vi "End Time.vi"(4 "Manual # of Averages":i32=1, 5 "Freq Index":i32, 6 "Signal Averages Selection":bool, 7 "Amp Index":i32, 8 "# of Pre-Check Points Collected (above 1 HZ)":i32=10, 9 "Np to Pre-Check (<1Hz)":i32=1, 10 "fp Array":dbl[](array[numeric]), 11 "# Amplitudes":i32) -> (3 "Estimated \nEnd Time":timestamp format="%<%I:%M:%S %p\n%x>T")   [LabVIEW 2018]
panel:
  # "Estimate time that NLEISRun sweep will end"
  # "Input"
  # "Output"
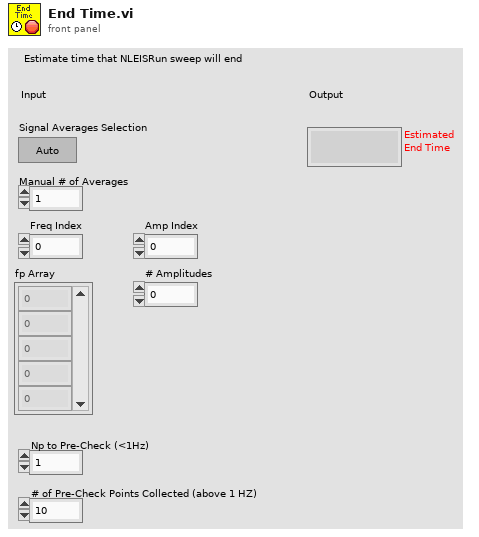
[diagram p1: front panel]
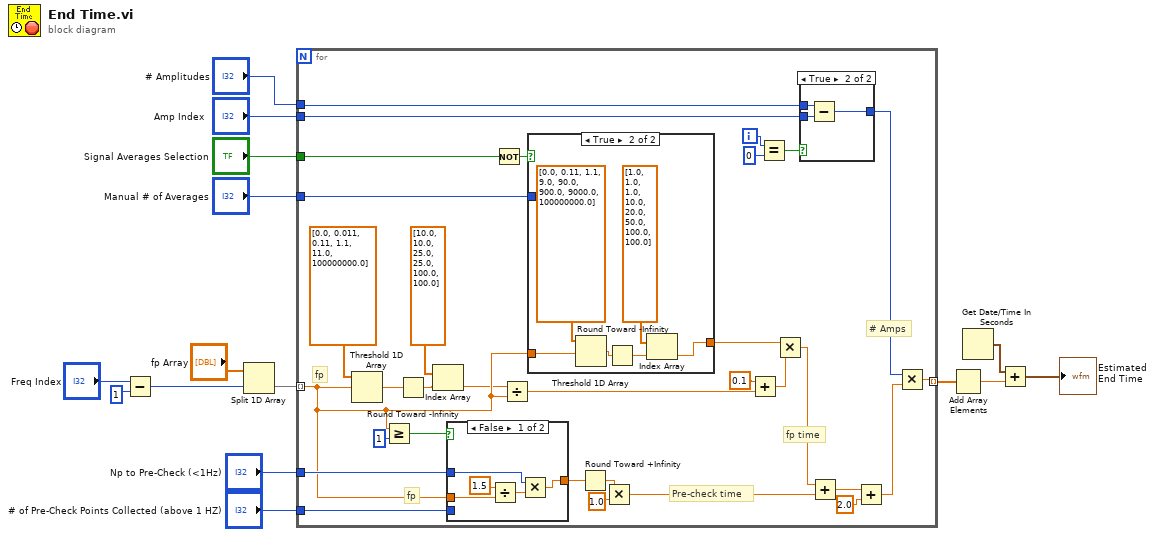
[diagram p0: block diagram]
diagram:
  n1 = Subtract(x="Freq Index", y=1) -> (x-y=w6:i32)
  n2 = Split 1D Array(array="fp Array", index=w6) -> (second subarray=w10:dbl[])  [unwired: 1 out]
  n3 = for {
    tunnel: w10 -> [w19] mode=indexing
    tunnel: "# Amplitudes" -> [w30]
    tunnel: "Amp Index" -> [w29]
    tunnel: [w26] -> w15 mode=indexing
    tunnel: "# of Pre-Check Points Collected (above 1 HZ)" -> [w41]
    tunnel: "Np to Pre-Check (<1Hz)" -> [w40]
    tunnel: "Manual # of Averages" -> [w17]
    tunnel: "Signal Averages Selection" -> [w16]
    i -> [w31]
    # "# Amps"
    # "fp time"
    # "Pre-check time"
    # "fp"
    # "fp"
    n4 = Threshold 1D Array(2:w19, 3:dbl[] [0.0, 0.011, 0.11, 1.1, 11.0, 100000000.0]) -> (0:w22:dbl)  [unwired: 1 in]
    n5 = Greater Or Equal?(x=w19, y=1) -> (x >= y?=w46:bool)
    n6 = Round Toward -Infinity(1:w22) -> (0:w23:dbl)
    n7 = Index Array(array=dbl[] [10.0, 10.0, 25.0, 25.0, 100.0, 100.0], index=w23) -> (element=w18:dbl)
    n8 = case shown="False" w46 {
      tunnel: [w61 w64] -> w25
      tunnel: w19 -> [w60 _]
      tunnel: w41 -> [_ w64]
      tunnel: w40 -> [w59 _]
      frame False {
        n9 = Divide(x=1.5, y=w60) -> (x/y=w62:dbl)
        n10 = Multiply(x=w59, y=w62) -> (x*y=w61:dbl)
      }
      frame True {
      }
    }
    n11 = Not(x=w16) -> (.not. x?=w39:bool)
    n12 = Divide(x=w18, y=w19) -> (x/y=w36:dbl)
    n13 = case shown="True" w39 {
      tunnel: [w52 w54] -> w38
      tunnel: w19 -> [_ w53]
      tunnel: w17 -> [w52 _]
      frame False {
      }
      frame True {
        n14 = Threshold 1D Array(2:w53, 3:dbl[] [0.0, 0.11, 1.1, 9.0, 90.0, 900.0, 9000.0, 100000000.0]) -> (0:w57:dbl)  [unwired: 1 in]
        n15 = Round Toward -Infinity(1:w57) -> (0:w58:dbl)
        n16 = Index Array(array=dbl[] [1.0, 1.0, 1.0, 10.0, 20.0, 50.0, 100.0, 100.0], index=w58) -> (element=w54:dbl)
      }
    }
    n17 = Round Toward +Infinity(x=w25) -> (ceil(x): smallest int >= x=w24:dbl)
    n18 = Multiply(x=w24, y=1.0 ("x")) -> (x*y=w44:dbl)
    n19 = Add(x=0.1, y=w36) -> (x+y=w37:dbl)
    n20 = Equal?(x=w31, y=0) -> (x = y?=w33:bool)
    n21 = Multiply(x=w38, y=w37) -> (x*y=w34:dbl)
    n22 = case shown="True" w33 {
      tunnel: w30 -> [w48 w51]
      tunnel: [w48 w50] -> w28
      tunnel: w29 -> [_ w49]
      frame False {
      }
      frame True {
        n23 = Subtract(x=w51, y=w49) -> (x-y=w50:i32)
      }
    }
    n24 = Add(x=w34, y=w44) -> (x+y=w43:dbl)
    n25 = Add(x=w43, y=2.0 ("x")) -> (x+y=w27:dbl)
    n26 = Multiply(x=w28, y=w27) -> (x*y=w26:dbl)
  }
  n27 = Add Array Elements(numeric array=w15) -> (sum=w14:dbl)
  n28 = Get Date/Time In Seconds() -> (seconds since 1Jan1904=w13:timestamp)
  n29 = Add(x=w13, y=w14) -> (x+y=→"Estimated \nEnd Time":timestamp)
